vi "Calibrate filter wheel.vi"(8 "Error In":errorcluster) -> (0 "error out":errorcluster, 1 "Rotation time (ms)":dbl, 2 "Enable Channel out":u8=11, 3 "Serial Port out":refnum<visa-resource-name>="COM3", 4 "No of points":i32, 5 "VISA resource name out":refnum<visa-resource-name>)   [LabVIEW 2011]
uses:
  <vilib>/MakerHub/LINX/Public/Peripherals/Digital/Digital Write 1 Chan.vi
  <vilib>/MakerHub/LINX/LMH-LINX.lvlib
  <instrlib>/keithley_24xx/Keithley 24XX/Keithley 24XX.lvlib
panel:
  in  "Angle (degrees)":dbl=360.0
  in  "Clockwise?":bool=TRUE
  in  "Enable Channel":u8=11
  in  "Direction Channel":u8=8
  in  "Step Channel":u8=9
  in  "Serial Port":refnum<visa-resource-name>="COM3"
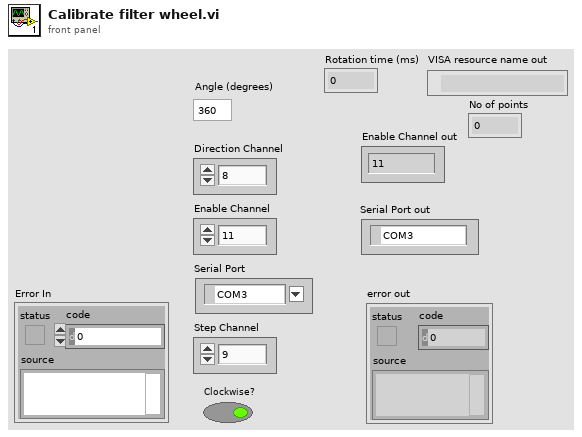
[diagram p1: front panel]
types:
  T1 = typedef "LMH-LINX.lvlib/LINX Ref.ctl" = cluster{"Platform":T2, "Interface":T3, "LINX Device Config":T4}
  T2 = typedef "LMH-LINX.lvlib/Platform.ctl" = enum16{"LINX", "myRIO"}
  T3 = typedef "LMH-LINX.lvlib/Interface.ctl" = enum16{"Serial", "TCP"}
  T4 = typedef "LMH-LINX.lvlib/Device.lvlib/LINX Device Config.ctl" = cluster{"Interface":T3, "COM Port":refnum<visa-resource-name>, "TCP Configuration":T5, "Device Family":u8, "Device ID":u8, "Device Name":string, "TCP Ref":refnum<k5>, "Channels":T6}
  T5 = typedef "LMH-LINX.lvlib/Device.lvlib/TCP Config.ctl" = cluster{"IP Address":string, "Port":u16}
  T6 = typedef "LMH-LINX.lvlib/Channels.ctl" = cluster{"DI":u8[], "DO":u8[], "AI":u8[], "AO":u8[], "PWM":u8[], "QE":u8[], "UART":u8[], "I2C 2":u8[], "SPI":u8[], "CAN":u8[], "Servo":u8[], "AI Ref (V)":dbl, "AO Ref (V)":dbl, "AO Resolution (Bits)":u8}
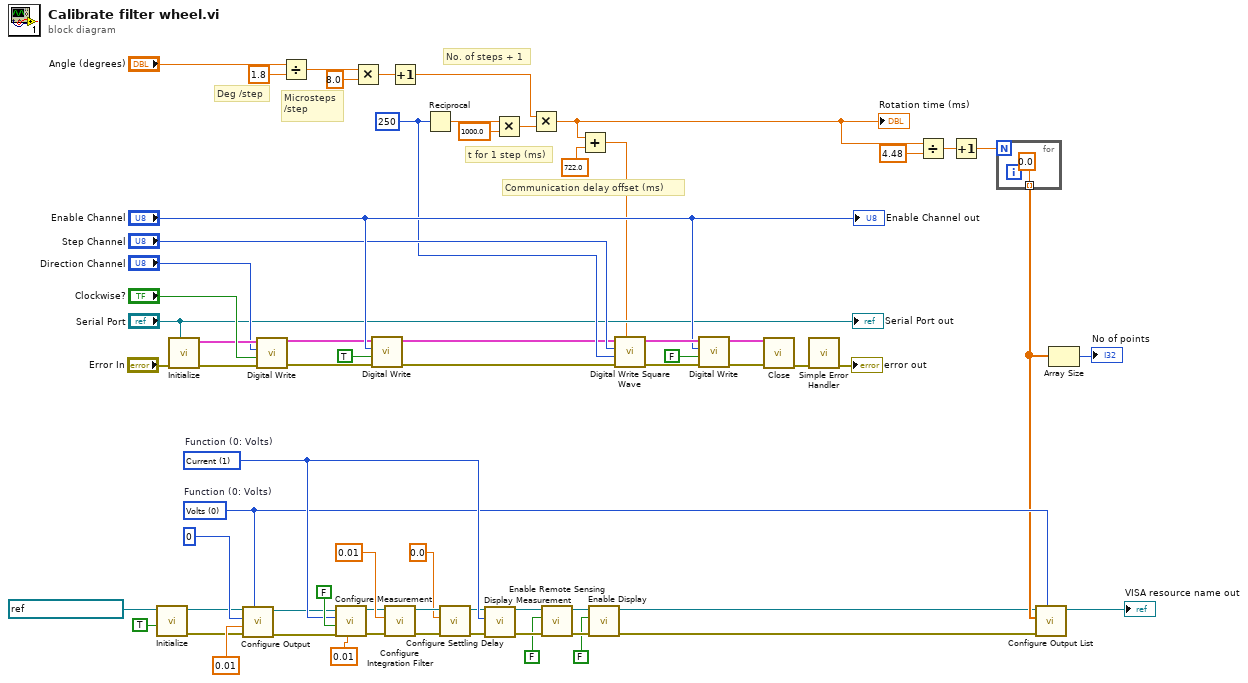
[diagram p0: block diagram]
diagram:
  w17 = u16 0 items=["Volts", "Current", "Resistance"]  # Function (0: Volts)
  w36 = u16 1 items=["Volts", "Current", "Resistance"]  # Function (0: Volts)
  w10 = u32 250 ("Frequency (Hz)")
  # "Communication delay offset (ms)"
  # "t for 1 step (ms)"
  # "No. of steps + 1"
  # "Microsteps\n/step"
  # "Deg /step"
  n1 = call <instrlib>:"Initialize.vi"("Reset (True)"=TRUE, "VISA resource name"=refnum<visa-resource-name> "GPIB0::24::INSTR") -> ("error out"=w20:errorcluster, "VISA resource name out"=w21:refnum<visa-resource-name>)  [unwired: 3 in, 5 out]
  n2 = call <instrlib>:"Initialize.vi"("Serial Port"="Serial Port", "Error In"="Error In") -> ("Error Out"=w57:errorcluster, "LINX Ref"=w58:T1)  [unwired: 7 in, 1 out]
  n3 = call <instrlib>:"Configure Output.vi"("Source Mode  (0: Voltage)"=w17, "error in (no error)"=w20, "Compliance  Level (0.1)"=0.01 ("Compliance  Level"), "Output Level (0)"=0, "VISA resource name"=w21) -> ("error out"=w18:errorcluster, "VISA resource name out"=w19:refnum<visa-resource-name>)  [unwired: 5 in]
  n4 = call-poly <vilib>:"Digital Write.vi"("Error In"=w57, "Output Value"="Clockwise?", "DO Channel"="Direction Channel", "LINX Resource"=w58) -> ("Error Out"=w52:errorcluster, "LINX Resource"=w53:T1)  [unwired: 6 in]
  n5 = Divide(x="Angle (degrees)", y=1.8) -> (x/y=w49:dbl)
  n6 = call <instrlib>:"Configure Measurement.vi"("Manual Range (1.0)"=0.01, "error in (no error)"=w18, "Enable Auto Range (T:Enable)"=FALSE, "Function (0: Volts)"=w36, "VISA resource name"=w19) -> ("error out"=w31:errorcluster, "VISA resource name out"=w30:refnum<visa-resource-name>)  [unwired: 5 in]
  n7 = Multiply(x=w49, y=8.0) -> (x*y=w44:dbl)
  n8 = call-poly <vilib>:"Digital Write.vi"("Error In"=w52, "Output Value"=TRUE ("LED Value"), "DO Channel"="Enable Channel", "LINX Resource"=w53) -> ("Error Out"=w7:errorcluster, "LINX Resource"=w8:T1)  [unwired: 6 in]
  n9 = call <instrlib>:"Configure Integration Filter.vi"("error in (no error)"=w31, "Measurement Speed (1 PLC)"=0.01, "VISA resource name"=w30) -> ("error out"=w38:errorcluster, "VISA resource name out"=w37:refnum<visa-resource-name>)  [unwired: 7 in]
  n10 = Increment(x=w44) -> (x+1=w43:dbl)
  n11 = Reciprocal(x=w10) -> (1/x=w47:dbl)
  n12 = call <instrlib>:"Configure Settling Delay.vi"("error in (no error)"=w38, "Manual Settling Delay (0 sec)"=0.0, "VISA resource name"=w37) -> ("error out"=w35:errorcluster, "VISA resource name out"=w34:refnum<visa-resource-name>)  [unwired: 7 in]
  n13 = call <instrlib>:"Display Measurement.vi"("error in (no error)"=w35, "Displayed Measurement (0: Voltage)"=w36, "VISA resource name"=w34) -> ("error out"=w33:errorcluster, "VISA resource name out"=w32:refnum<visa-resource-name>)  [unwired: 7 in]
  n14 = Multiply(x=w47, y=1000.0) -> (x*y=w45:dbl)
  n15 = Multiply(x=w43, y=w45) -> (x*y=w5:dbl)
  "Rotation time (ms)" <- w5
  n16 = call <instrlib>:"Enable Remote Sensing.vi"("error in (no error)"=w33, "Enable Remote Sensing (T: Enable)"=FALSE, "VISA resource name"=w32) -> ("error out"=w28:errorcluster, "VISA resource name out"=w29:refnum<visa-resource-name>)  [unwired: 7 in]
  n17 = Add(x=w5, y=722.0) -> (x+y=w4:dbl)
  n18 = call <instrlib>:"Enable Display.vi"("error in (no error)"=w28, "Enable Display (T: Enable)"=FALSE ("Enable Output (T: Enable)"), "VISA resource name"=w29) -> ("error out"=w2:errorcluster, "VISA resource name out"=w3:refnum<visa-resource-name>)  [unwired: 7 in]
  n19 = call <vilib>:"Digital Write Square Wave.vi"("Duration (ms)"=w4, "Error In"=w7, "Frequency (Hz)"=w10, "Channel"="Step Channel", "LINX Resource"=w8) -> ("Error Out"=w64:errorcluster, "LINX Resource"=w65:T1)  [unwired: 5 in]
  n20 = call-poly <vilib>:"Digital Write.vi"("Error In"=w64, "Output Value"=FALSE ("LED Value"), "DO Channel"="Enable Channel", "LINX Resource"=w65) -> ("Error Out"=w61:errorcluster, "LINX Resource"=w62:T1)  [unwired: 6 in]
  n21 = call <vilib>:"Close.vi"("Error In"=w61, "LINX Resource"=w62) -> ("Error Out"=w67:errorcluster)  [unwired: 8 in, 1 out]
  n22 = call <vilib>:"Simple Error Handler.vi"("error in (no error)"=w67) -> ("error out"=→"error out":errorcluster)  [unwired: 4 in, 4 out]
  n23 = Divide(x=w5, y=4.48) -> (x/y=w16:dbl)
  n24 = Increment(x=w16) -> (x+1=w15:dbl)
  n25 = for {
    N: w15 -> [_]
    tunnel: [0.0 ("y")] -> w14 mode=indexing
  }
  n26 = call <instrlib>:"Configure Output List.vi"("Source Mode  (0: Voltage)"=w17, "error in (no error)"=w2, "Output List"=w14, "VISA resource name"=w3) -> ("VISA resource name out"=→"VISA resource name out":refnum<visa-resource-name>)  [unwired: 6 in, 1 out]
  n27 = Array Size(array=w14) -> (size(s)=→"No of points":i32)
  "Serial Port out" <- "Serial Port"
  "Enable Channel out" <- "Enable Channel"
